vi "Decode status bit.vi"(3 "Values":dbl[](array[numeric]) format="%.6f", 4 "Bit to check for":i32) -> (17 "Decoded bit":bool[](array[boolean]))   [LabVIEW 2026]
doc: "This VI checks the status bit value for a certain bit and returns Decoded_bit indicating whether that bit has a value of TRUE or FALSE."
panel:
  # "This vi checks the status bit value for a certain bit and returns \n\"Decoded bit\" indicating whether that bit has a value of TRUE or FALSE."
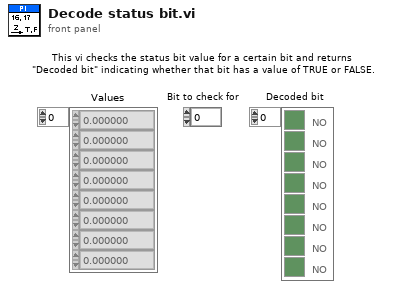
[diagram p1: front panel]
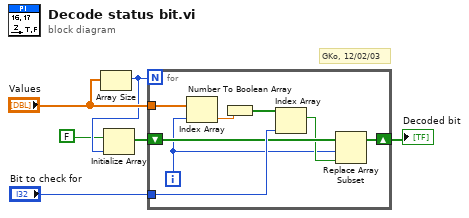
[diagram p0: block diagram]
diagram:
  # "GKo, 12/02/03"
  n1 = Array Size(array="Values") -> (size(s)=w4:i32)
  n2 = Initialize Array(FALSE, w4) -> (w2:bool[])
  n3 = for {
    N: w4 -> [_]
    shift-right: [w7] -> w5
    shift-left: w2 -> [w10]
    tunnel: "Values" -> [w14]
    tunnel: "Bit to check for" -> [w11]
    i -> [w8]
    n4 = Index Array(array=w14, index=w8) -> (element=w13:dbl)
    n5 = Number To Boolean Array(number=w13) -> (Boolean array=w12:bool[])
    n6 = Index Array(array=w12, index=w11) -> (element=w9:bool)
    n7 = Replace Array Subset(array=w10, new element=w9, index=w8) -> (w7:bool[])
  }
  "Decoded bit" <- w5
